vi "Close_Instr.vi"(8 "error in (no error)":errorcluster caption="entrée d'erreur (pas d'erreur)", 11 "Class Relay_Board en entrée":refnum<class "Class Instrument Relay_Board.lvclass">) -> (0 "error out":errorcluster caption="sortie d'erreur", 3 "Class Relay_Board en Sortie":refnum<class "Class Instrument Relay_Board.lvclass">)   [LabVIEW 2020, in "Library Instrument & Equipement.lvlib" / "Library Instruments.lvlib" / "Class Instrument Relay_Board.lvclass"]
uses:
  Class Instrument Relay_Board.lvclass
  Class Instrument Relay_Board.lvclass/Class Instrument Relay_Board.ctl
  Relay_Board/Relay_Board (Default)/Class Relay_Board (Default).lvclass
  Instrument (Default)/Class Instrument (Default).lvclass
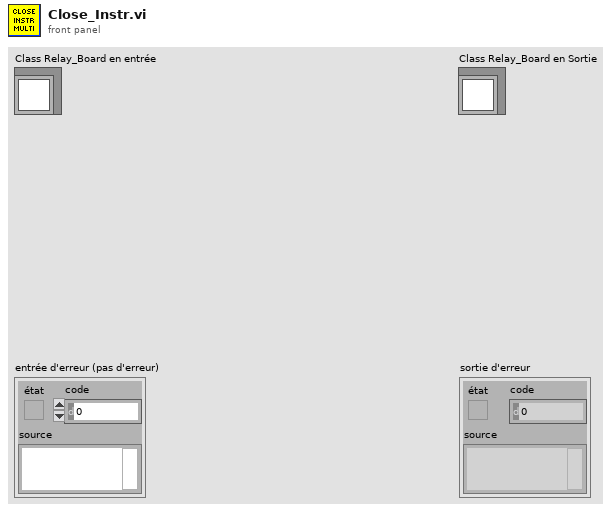
[diagram p1: front panel]
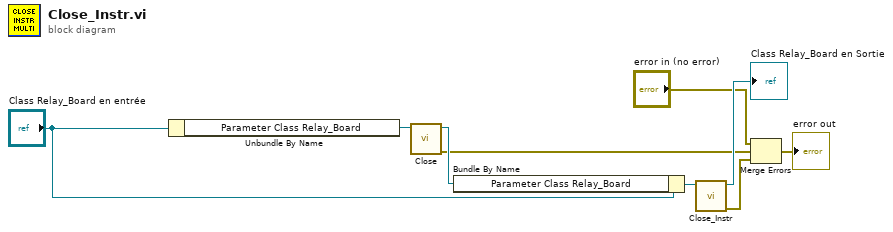
[diagram p0: block diagram]
diagram:
  n1 = Unbundle By Name("Class Relay_Board en entrée") -> ("Parameter Class Relay_Board"=w8:refnum<class "Class Relay_Board (Default).lvclass">)
  n2 = call-dynamic "Close.vi"("Class Relay_Board (Default) en entrée"=w8) -> ("error out"=w2:errorcluster, "Class Relay_Board (Default) en sortie"=w7:refnum<class "Class Relay_Board (Default).lvclass">)  [unwired: 9 in]
  n3 = Bundle By Name(cluster="Class Relay_Board en entrée", "Parameter Class Relay_Board"=w7) -> (w5:refnum<class "Class Instrument Relay_Board.lvclass">)
  n4 = call-parent "Close_Instr.vi"("Class Instrument (Default) en entrée"=w5) -> ("error out"=w3:errorcluster, "Class Instrument (Default) en sortie"=→"Class Relay_Board en Sortie":refnum<class "Class Instrument Relay_Board.lvclass">)  [unwired: 9 in]
  n5 = Merge Errors("error in (no error)", w2, w3) -> (→"error out":errorcluster)
